vi "Ex7_Feu_Signialisation.vi"() -> ()   [LabVIEW 2018]
uses:
  Ex7_Feu_Signialisation_Var_1.vi
panel:
  in  "stop":bool
  out "Vert":bool
  out "Jaune":bool
  out "Rouge":bool
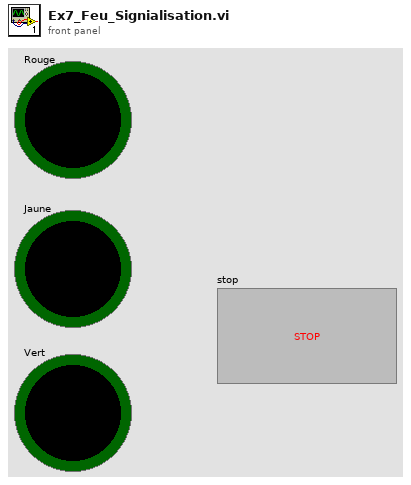
[diagram p1: front panel]
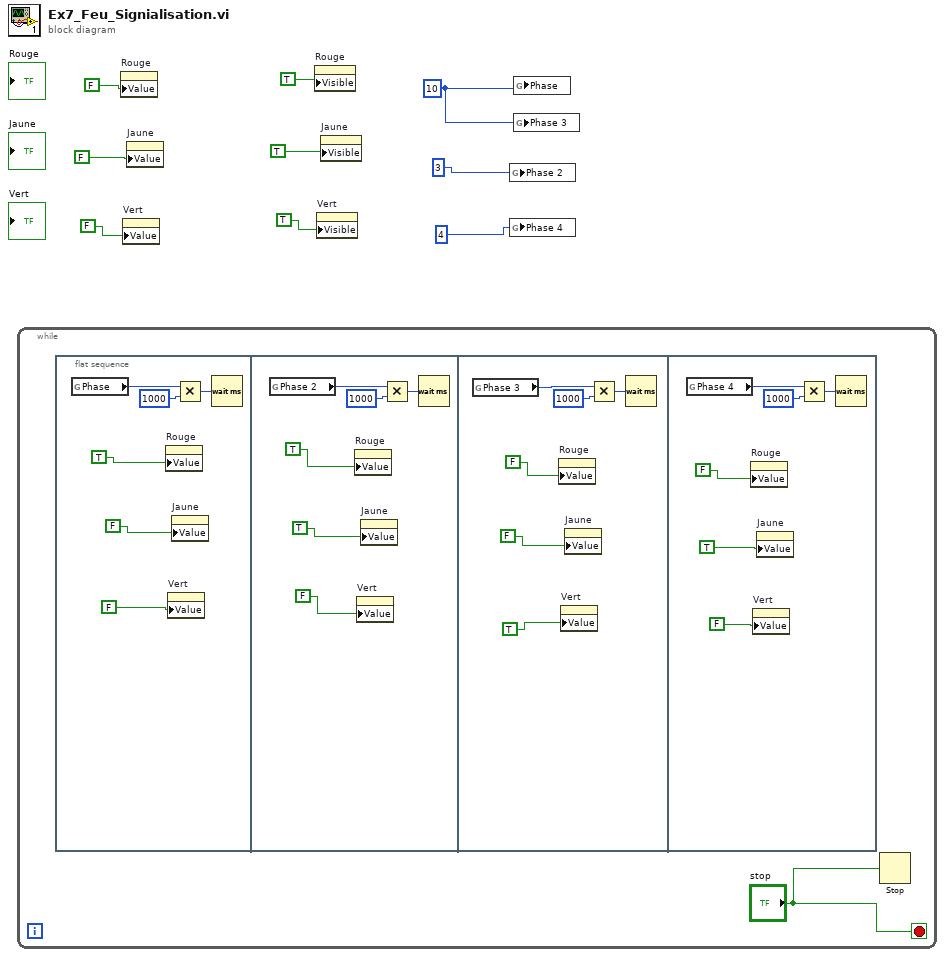
[diagram p0: block diagram]
diagram:
  w3 = u64 10 ("Phase 3")
  n1 = while {
    stop <- "stop" stop-if-true
    n2 = flat-sequence {
      frame #0 {
        n3 = global read "Ex7_Feu_Signialisation_Var_1.vi" "Phase"() -> (w16:u64)
        n4 = property on="Rouge" class="Bool (strict)"("Value"=TRUE) -> ()  [unwired: 2 in, 2 out]
        n5 = property on="Vert" class="Bool (strict)"("Value"=FALSE) -> ()  [unwired: 2 in, 2 out]
        n6 = property on="Jaune" class="Bool (strict)"("Value"=FALSE) -> ()  [unwired: 2 in, 2 out]
        n7 = Multiply(x=w16, y=u64 1000) -> (x*y=w14:u64)
        n8 = Wait (ms)(milliseconds to wait=w14) -> ()  [unwired: 1 out]
      }
      frame #1 {
        n9 = global read "Ex7_Feu_Signialisation_Var_1.vi" "Phase 2"() -> (w21:u64)
        n10 = property on="Rouge" class="Bool (strict)"("Value"=TRUE) -> ()  [unwired: 2 in, 2 out]
        n11 = property on="Vert" class="Bool (strict)"("Value"=FALSE) -> ()  [unwired: 2 in, 2 out]
        n12 = property on="Jaune" class="Bool (strict)"("Value"=TRUE) -> ()  [unwired: 2 in, 2 out]
        n13 = Multiply(x=w21, y=u64 1000) -> (x*y=w20:u64)
        n14 = Wait (ms)(milliseconds to wait=w20) -> ()  [unwired: 1 out]
      }
      frame #2 {
        n15 = global read "Ex7_Feu_Signialisation_Var_1.vi" "Phase 3"() -> (w27:u64)
        n16 = property on="Rouge" class="Bool (strict)"("Value"=FALSE) -> ()  [unwired: 2 in, 2 out]
        n17 = property on="Vert" class="Bool (strict)"("Value"=TRUE) -> ()  [unwired: 2 in, 2 out]
        n18 = property on="Jaune" class="Bool (strict)"("Value"=FALSE) -> ()  [unwired: 2 in, 2 out]
        n19 = Multiply(x=w27, y=u64 1000) -> (x*y=w26:u64)
        n20 = Wait (ms)(milliseconds to wait=w26) -> ()  [unwired: 1 out]
      }
      frame #3 {
        n21 = global read "Ex7_Feu_Signialisation_Var_1.vi" "Phase 4"() -> (w33:u64)
        n22 = property on="Rouge" class="Bool (strict)"("Value"=FALSE) -> ()  [unwired: 2 in, 2 out]
        n23 = property on="Vert" class="Bool (strict)"("Value"=FALSE) -> ()  [unwired: 2 in, 2 out]
        n24 = property on="Jaune" class="Bool (strict)"("Value"=TRUE) -> ()  [unwired: 2 in, 2 out]
        n25 = Multiply(x=w33, y=u64 1000) -> (x*y=w32:u64)
        n26 = Wait (ms)(milliseconds to wait=w32) -> ()  [unwired: 1 out]
      }
    }
    n27 = Stop(stop? (T)="stop") -> ()
  }
  n28 = property on="Rouge" class="Bool (strict)"("Value"=FALSE) -> ()  [unwired: 2 in, 2 out]
  n29 = property on="Vert" class="Bool (strict)"("Value"=FALSE) -> ()  [unwired: 2 in, 2 out]
  n30 = property on="Jaune" class="Bool (strict)"("Value"=FALSE) -> ()  [unwired: 2 in, 2 out]
  n31 = property on="Rouge" class="Bool (strict)"("Visible"=TRUE) -> ()  [unwired: 2 in, 2 out]
  n32 = property on="Vert" class="Bool (strict)"("Visible"=TRUE) -> ()  [unwired: 2 in, 2 out]
  n33 = property on="Jaune" class="Bool (strict)"("Visible"=TRUE) -> ()  [unwired: 2 in, 2 out]
  n34 = global write "Ex7_Feu_Signialisation_Var_1.vi" "Phase 2"(u64 3 ("Phase 3")) -> ()
  n35 = global write "Ex7_Feu_Signialisation_Var_1.vi" "Phase 4"(u64 4 ("Phase 3")) -> ()
  n36 = global write "Ex7_Feu_Signialisation_Var_1.vi" "Phase"(w3) -> ()
  n37 = global write "Ex7_Feu_Signialisation_Var_1.vi" "Phase 3"(w3) -> ()
